vi "SE_HV200.ProcEvents.vi"(0 "i ref in":refnum<vi>, 5 "error in":errorcluster) -> (14 "i ref out":refnum<vi>, 19 "error out":errorcluster)   [LabVIEW 2014, in "SE_HV200.lvlib"]
doc: "This method is used to define the events the object will listen to. Add your own events here."
uses:
  SE_HV200.lvlib
  CSCore/BaseProcess/BaseProcess.event definition.ctl
  CSCore/CAEObj/CAEObj.event definition.ctl
  CSCore/BaseProcess/BaseProcess.descriptor string definition.ctl
  CSCore/BaseProcess/BaseProcess.lvlib
  CSCore/CAEObj/CAEObj.lvlib
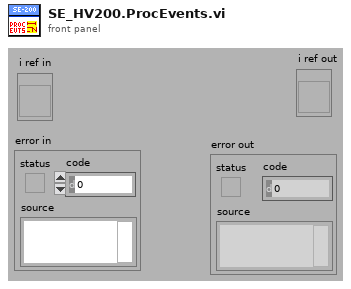
[diagram p1: front panel]
types:
  T1 = typedef "BaseProcess.lvlib/BaseProcess.event definition.ctl" = cluster{"CAEEvtDef":T2, "Data Descriptor":T3}
  T2 = typedef "CAEObj.lvlib/CAEObj.event definition.ctl" = cluster{"URL":string, "enable":bool, "ignoreResID":bool}
  T3 = typedef "BaseProcess.lvlib/BaseProcess.descriptor string definition.ctl" = string
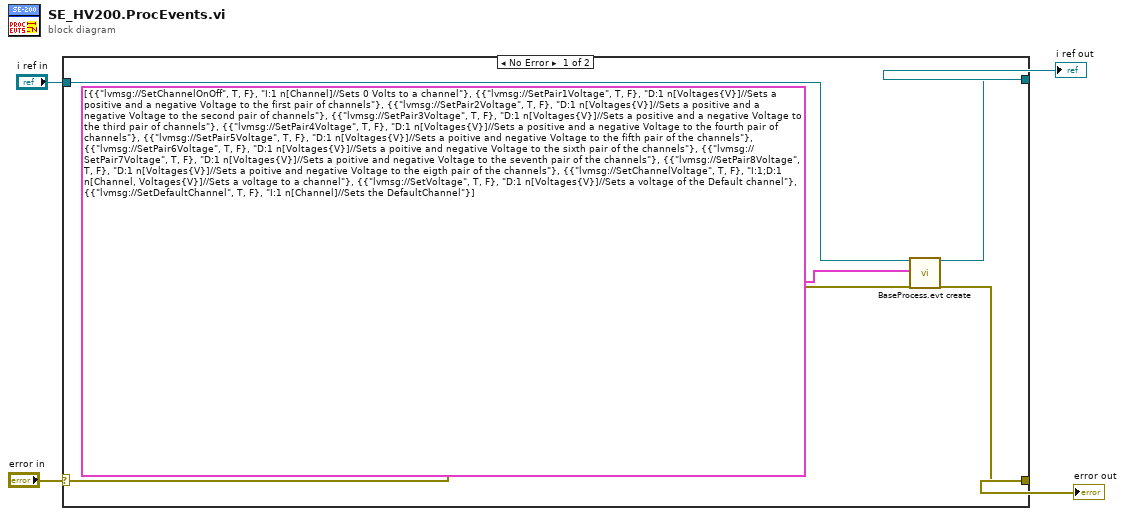
[diagram p0: block diagram]
diagram:
  n1 = case shown="No Error" "error in" {
    selector: "error in" -> [w5 w11]
    tunnel: "i ref in" -> [w9 w10]
    tunnel: [w8 w11] -> w3
    tunnel: [w7 w10] -> w2
    frame No Error {
      n2 = call "BaseProcess.evt create.vi"("i ref in"=w9, "newEvents"=T1[] [{"CAEEvtDef"={"URL"="lvmsg://SetChannelOnOff", "enable"=TRUE, "ignoreResID"=FALSE}, "Data Descriptor"="I:1 n[Channel]//Sets 0 Volts to a channel"}, {"CAEEvtDef"={"URL"="lvmsg://SetPair1Voltage", "enable"=TRUE, "ignoreResID"=FALSE}, "Data Descriptor"="D:1 n[Voltages{V}]//Sets a positive and a negative Voltage to the first pair of channels"}, {"CAEEvtDef"={"URL"="lvmsg://SetPair2Voltage", "enable"=TRUE, "ignoreResID"=FALSE}, "Data Descriptor"="D:1 n[Voltages{V}]//Sets a positive and a negative Voltage to the second pair of channels"}, {"CAEEvtDef"={"URL"="lvmsg://SetPair3Voltage", "enable"=TRUE, "ignoreResID"=FALSE}, "Data Descriptor"="D:1 n[Voltages{V}]//Sets a positive and a negative Voltage to the third pair of channels"}, {"CAEEvtDef"={"URL"="lvmsg://SetPair4Voltage", "enable"=TRUE, "ignoreResID"=FALSE}, "Data Descriptor"="D:1 n[Voltages{V}]//Sets a positive and a negative Voltage to the fourth pair of channels"}, {"CAEEvtDef"={"URL"="lvmsg://SetPair5Voltage", "enable"=TRUE, "ignoreResID"=FALSE}, "Data Descriptor"="D:1 n[Voltages{V}]//Sets a poitive and negative Voltage to the fifth pair of the channels"}, {"CAEEvtDef"={"URL"="lvmsg://SetPair6Voltage", "enable"=TRUE, "ignoreResID"=FALSE}, "Data Descriptor"="D:1 n[Voltages{V}]//Sets a poitive and negative Voltage to the sixth pair of the channels"}, {"CAEEvtDef"={"URL"="lvmsg://SetPair7Voltage", "enable"=TRUE, "ignoreResID"=FALSE}, "Data Descriptor"="D:1 n[Voltages{V}]//Sets a poitive and negative Voltage to the seventh pair of the channels"}, {"CAEEvtDef"={"URL"="lvmsg://SetPair8Voltage", "enable"=TRUE, "ignoreResID"=FALSE}, "Data Descriptor"="D:1 n[Voltages{V}]//Sets a poitive and negative Voltage to the eigth pair of the channels"}, {"CAEEvtDef"={"URL"="lvmsg://SetChannelVoltage", "enable"=TRUE, "ignoreResID"=FALSE}, "Data Descriptor"="I:1;D:1 n[Channel, Voltages{V}]//Sets a voltage to a channel"}, {"CAEEvtDef"={"URL"="lvmsg://SetVoltage", "enable"=TRUE, "ignoreResID"=FALSE}, "Data Descriptor"="D:1 n[Voltages{V}]//Sets a voltage of the Default channel"}, {"CAEEvtDef"={"URL"="lvmsg://SetDefaultChannel", "enable"=TRUE, "ignoreResID"=FALSE}, "Data Descriptor"="I:1 n[Channel]//Sets the DefaultChannel"}] ("new events"), "error in (no error)"=w5) -> ("i ref out"=w7:refnum<vi>, "error out"=w8:errorcluster)  [unwired: 13 in, 2 out]
    }
    frame Error {
    }
  }
  "i ref out" <- w2
  "error out" <- w3
